vi "TDC Globals.vi"() -> ()   [LabVIEW 2015, in "ECS-RT.lvlib"]
uses:
  ECS-RT.lvlib
panel:
  in  "ESTTL2-8_TDC":sgl
  in  "ESTTL2-7_TDC":sgl
  in  "ESTTL2-6_TDC":sgl
  in  "ESTTL2-5_TDC":sgl
  in  "ESTTL2-4_TDC":sgl
  in  "ESTTL2-3_TDC":sgl
  in  "ESTTL2-2_TDC":sgl
  in  "ESTTL2-1_TDC":sgl
  in  "Global TDC Offset (CAD)":sgl
  in  "VVT_TDCRef":sgl
  in  "DI4-2_Order":i32
  in  "DI4-1_Order":i32
  in  "DI3-2_Order":i32
  in  "DI3-1_Order":i32
  in  "DI2-2_Order":i32
  in  "DI2-1_Order":i32
  in  "DI1-2_Order":i32
  in  "DI1-1_Order":i32
  in  "PFI2-4_TDC":sgl
  in  "PFI2-3_TDC":sgl
  in  "PFI2-2_TDC":sgl
  in  "PFI2-1_TDC":sgl
  in  "PFI1-4_TDC":sgl
  in  "PFI1-3_TDC":sgl
  in  "PFI1-2_TDC":sgl
  in  "PFI1-1_TDC":sgl
  in  "ESTTL1-8_TDC":sgl
  in  "ESTTL1-7_TDC":sgl
  in  "ESTTL1-6_TDC":sgl
  in  "ESTTL1-5_TDC":sgl
  in  "ESTTL1-4_TDC":sgl
  in  "ESTTL1-3_TDC":sgl
  in  "ESTTL1-2_TDC":sgl
  in  "ESTTL1-1_TDC":sgl
  in  "DI4-2_TDC":sgl
  in  "DI4-1_TDC":sgl
  in  "DI3-2_TDC":sgl
  in  "DI3-1_TDC":sgl
  in  "DI2-2_TDC":sgl
  in  "DI2-1_TDC":sgl
  in  "DI1-2_TDC":sgl
  in  "DI1-1_TDC":sgl
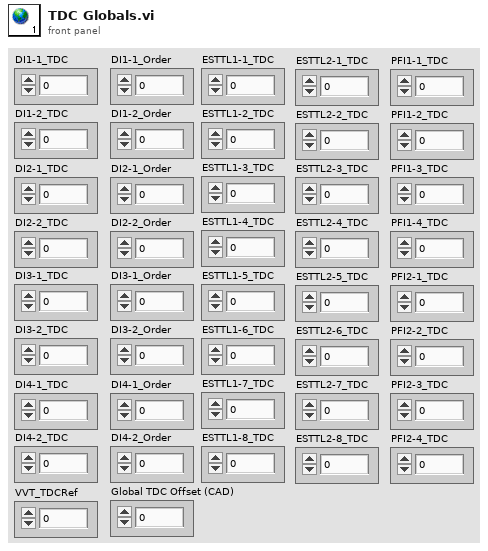
[diagram p1: front panel]
diagram:
